vi "Update Graphs.vi"(8 "error in (no error)":errorcluster, 10 "image":variant[][](array[variant]), 11 "Detail Graph in":refnum<class "Detail Graph.lvclass">) -> (0 "error out":errorcluster, 1 "Cursor.Cursor Position":T1, 3 "Detail Graph out":refnum<class "Detail Graph.lvclass">)   [LabVIEW 2023, in "Detail Graph.lvclass"]
uses:
  Detail Graph.lvclass
  <vilib>/Utility/miscctls.llb/LVPointDoubleTypeDef.ctl
  Base Graph/Base Graph.lvclass/Base Graph.ctl
  Detail Graph.lvclass/Detail Graph.ctl
  Base Graph/Base Graph.lvclass
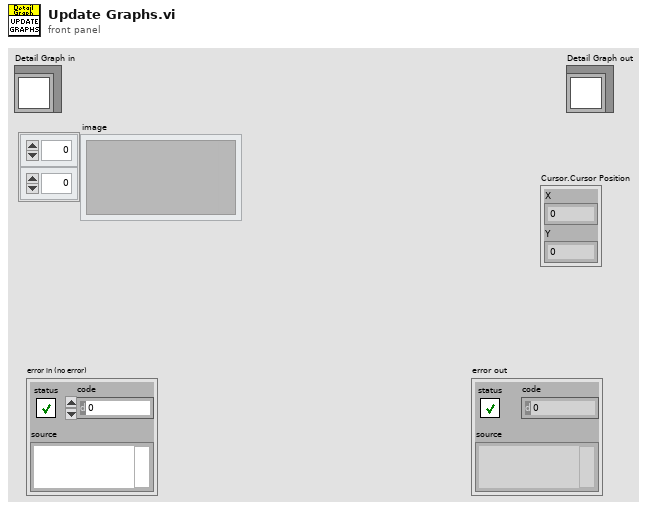
[diagram p1: front panel]
types:
  T1 = typedef "LVPointDoubleTypeDef.ctl" = cluster{"X":dbl, "Y":dbl}
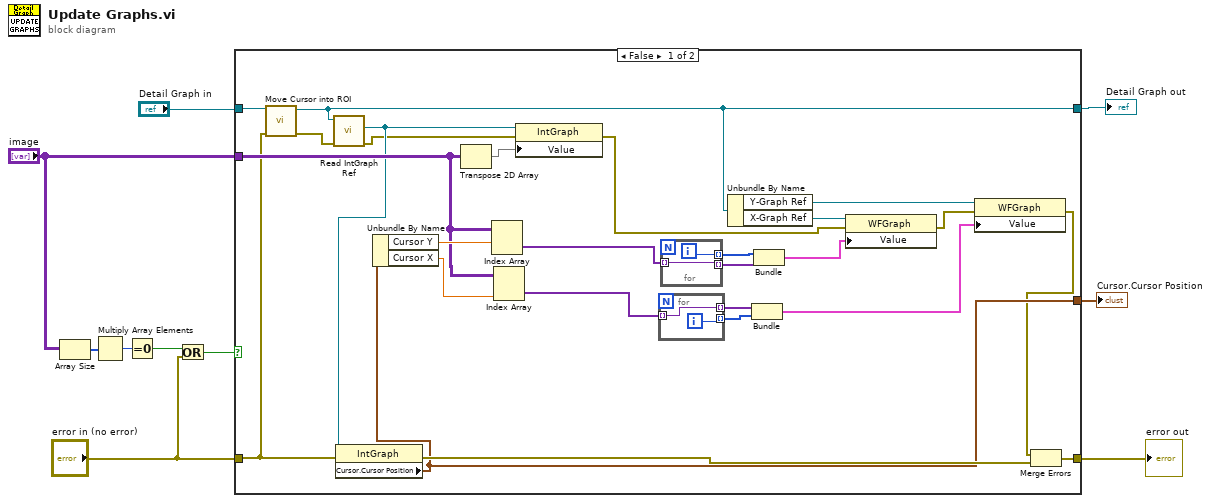
[diagram p0: block diagram]
diagram:
  n1 = Array Size(array="image") -> (size(s)=w5:i32[])
  n2 = Multiply Array Elements(1:w5) -> (0:w8:i32)
  n3 = Equal To 0?(x=w8) -> (x = 0?=w6:bool)
  n4 = Or(x=w6, y="error in (no error)") -> (x .or. y?=w7:bool)
  n5 = case shown="False" w7 {
    tunnel: [w16 w41] -> w10
    tunnel: [w21 w42] -> w2
    tunnel: "Detail Graph in" -> [w22 w42]
    tunnel: "image" -> [w32 _]
    tunnel: "error in (no error)" -> [w17 w41]
    tunnel: [w23 _] -> w1
    frame False {
      n6 = call "Move Cursor into ROI.vi"("error in (no error)"=w17, "Base Graph in"=w22) -> ("error out"=w20:errorcluster, "Base Graph out"=w21:refnum<class "Detail Graph.lvclass">)  [unwired: 8 in]
      n7 = call "Read IntGraph Ref.vi"("error in (no error)"=w20, "TG Base Graph in"=w21) -> ("error out"=w19:errorcluster, "IntGraph Ref"=w24:refnum<vi>)  [unwired: 7 in, 1 out]
      n8 = property class="IntGraph"(reference=w24, error in=w17) -> (error out=w25:errorcluster, "Cursor.Cursor Position"=w23:T1)  [unwired: 1 out]
      n9 = Unbundle By Name(w23) -> ("Cursor Y"=w35:dbl, "Cursor X"=w34:dbl)
      n10 = Transpose 2D Array(2D array=w32) -> (transposed array=w36:variant[][])
      n11 = Index Array(array=w32, index (row)=w35) -> (element=w12:variant[])  [unwired: 1 in]
      n12 = Index Array(array=w32, index (col)=w34) -> (element=w14:variant[])  [unwired: 1 in]
      n13 = property class="IntGraph"(reference=w24, error in=w19, "Value"=w36) -> (error out=w18:errorcluster)  [unwired: 1 out]
      n14 = for {
        tunnel: [w39] -> w33 mode=indexing
        tunnel: w14 -> [w40] mode=indexing
        tunnel: [w40] -> w13 mode=indexing
        i -> [w39]
      }
      n15 = for {
        tunnel: [w37] -> w26 mode=indexing
        tunnel: w12 -> [w38] mode=indexing
        tunnel: [w38] -> w11 mode=indexing
        i -> [w37]
      }
      n16 = Unbundle By Name(w21) -> ("Y-Graph Ref"=w31:refnum<vi>, "X-Graph Ref"=w29:refnum<vi>)
      n17 = Bundle(w13, w33) -> (w27:cluster{variant[], i32[]})  [unwired: 1 in]
      n18 = Bundle(w26, w11) -> (w28:cluster{i32[], variant[]})  [unwired: 1 in]
      n19 = property class="WFGraph"(reference=w29, error in=w18, "Value"=w28) -> (error out=w30:errorcluster)  [unwired: 1 out]
      n20 = property class="WFGraph"(reference=w31, error in=w30, "Value"=w27) -> (error out=w15:errorcluster)  [unwired: 1 out]
      n21 = Merge Errors(w15, w25) -> (w16:errorcluster)
    }
    frame True {
    }
  }
  "error out" <- w10
  "Detail Graph out" <- w2
  "Cursor.Cursor Position" <- w1
